vi "MotorSetup.vi"   [LabVIEW 2020]
uses:
  Swerve Global Variables.vi
types:
  T1 = typedef "WPI_MotorControlDeviceRef.ctl" = cluster{"DeviceStatus":errorcluster, "Type":T2, "PWM":cluster{"PWM Channel":T3, "DeadBand":T4}, "CAN":cluster{"Device Number":u8, "SetOutput VI Ref":variant, "GetOutput VI Ref":variant, "Enable VI Ref":variant, "Disable VI Ref":variant, "Data":variant}, "Invert":bool, "DIO PWM":cluster{"PWM \"Enable\" Channel":T3, "DIOChannel":T5, "PWM Rate":dbl}}
  T2 = typedef "WPI_MotorControlType.ctl" = enum16{"PWM", "CAN", "DIO PWM"}
  T3 = typedef "FPGA_DIOPWMChannel.ctl" = enum8{"PWM 0", "PWM 1", "PWM 2", "PWM 3", "PWM 4", "PWM 5", "PWM 6", "PWM 7", "PWM 8", "PWM 9", "PWM MXP 0", "PWM MXP 1", "PWM MXP 2", "PWM MXP 3", "PWM MXP 4", "PWM MXP 5", "PWM MXP 6", "PWM MXP 7", "PWM MXP 8", "PWM MXP 9", "Invalid"}
  T4 = typedef "WPI_PWMDeadband.ctl" = cluster{"Name":string, "maxPositivePwm":i32, "minPositivePwm":i32, "centerPwm":i32, "maxNegativePwm":i32, "minNegativePwm":i32, "angularRange":u16}
  T5 = typedef "FPGA_DIOChannel.ctl" = enum8{"DIO 0", "DIO 1", "DIO 2", "DIO 3", "DIO 4", "DIO 5", "DIO 6", "DIO 7", "DIO 8", "DIO 9", "DIO MXP 0", "DIO MXP 1", "DIO MXP 2", "DIO MXP 3", "DIO MXP 4", "DIO MXP 5", "DIO MXP 6", "DIO MXP 7", "DIO MXP 8", "DIO MXP 9", "DIO MXP 10", "DIO MXP 11", "DIO MXP 12", "DIO MXP 13", "DIO MXP 14", "DIO MXP 15", "SPI Port CS1", "SPI Port CS2", "SPI Port CS3", "SPI Port MISO", "SPI Port MOSI", "Invalid"}
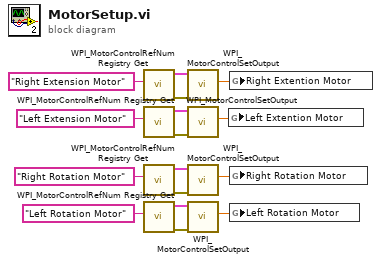
[diagram p0: block diagram]
diagram:
  n1 = call <vilib>:"WPI_MotorControlRefNum Registry Get.vi"("refnum name"="Right Extension Motor") -> ("error out"=w2:errorcluster, "MotorControlDevRef"=w1:T1)  [unwired: 9 in]
  n2 = call <vilib>:"WPI_MotorControlRefNum Registry Get.vi"("refnum name"="Left Extension Motor") -> ("error out"=w6:errorcluster, "MotorControlDevRef"=w5:T1)  [unwired: 9 in]
  n3 = call <vilib>:"WPI_MotorControlRefNum Registry Get.vi"("refnum name"="Right Rotation Motor") -> ("error out"=w10:errorcluster, "MotorControlDevRef"=w9:T1)  [unwired: 9 in]
  n4 = call <vilib>:"WPI_MotorControlRefNum Registry Get.vi"("refnum name"="Left Rotation Motor") -> ("error out"=w14:errorcluster, "MotorControlDevRef"=w13:T1)  [unwired: 9 in]
  n5 = call <vilib>:"WPI_MotorControlSetOutput.vi"("error in (no error)"=w2, "MotorControlDevRef"=w1) -> ("Motor Output"=w4:dbl)  [unwired: 7 in, 2 out]
  n6 = call <vilib>:"WPI_MotorControlSetOutput.vi"("error in (no error)"=w6, "MotorControlDevRef"=w5) -> ("Motor Output"=w8:dbl)  [unwired: 7 in, 2 out]
  n7 = call <vilib>:"WPI_MotorControlSetOutput.vi"("error in (no error)"=w10, "MotorControlDevRef"=w9) -> ("Motor Output"=w12:dbl)  [unwired: 7 in, 2 out]
  n8 = call <vilib>:"WPI_MotorControlSetOutput.vi"("error in (no error)"=w14, "MotorControlDevRef"=w13) -> ("Motor Output"=w16:dbl)  [unwired: 7 in, 2 out]
  n9 = global write "Swerve Global Variables.vi" "Left Extention Motor"(w8) -> ()
  n10 = global write "Swerve Global Variables.vi" "Right Extention Motor"(w4) -> ()
  n11 = global write "Swerve Global Variables.vi" "Right Rotation Motor"(w12) -> ()
  n12 = global write "Swerve Global Variables.vi" "Left Rotation Motor"(w16) -> ()
